vi "Voltage - Continuous Output.vi"() -> ()   [LabVIEW 2025]
doc: "This example demonstrates how to continuously re-generate analog output data from a buffer in your computer's memory.\n\nRefer to your device documentation for pinouts and hardware capabilities."
uses:
  <vilib>/Utility/error.llb/DialogType.ctl
  <vilib>/DAQmx/write.llb/DAQmx Write (Analog Wfm 1Chan NSamp).vi
  <vilib>/DAQmx/create/channels.llb/DAQmx Create Channel (AO-Voltage-Basic).vi
  <vilib>/DAQmx/configure/timing.llb/DAQmx Timing (Use Waveform).vi
  <vilib>/DAQmx/miscellaneous.llb/DAQmx Fill In Error Info.vi
panel:
  in  "Stop":bool
  out "Waveform Graph":waveform(dbl)(graph)
  in  "Max Voltage":dbl=5.0
  in  "Min Voltage":dbl=-5.0
  in  "Physical Channel(s)":tag="Dev1/ao0"
  # "Channel Settings"
  # "Output"
  # "Timing and\nBuffer Settings"
  # "Waveform Settings"
  # "The number of elements in the waveform array must equal the number of channels in the task."
  # "Trigger Settings"
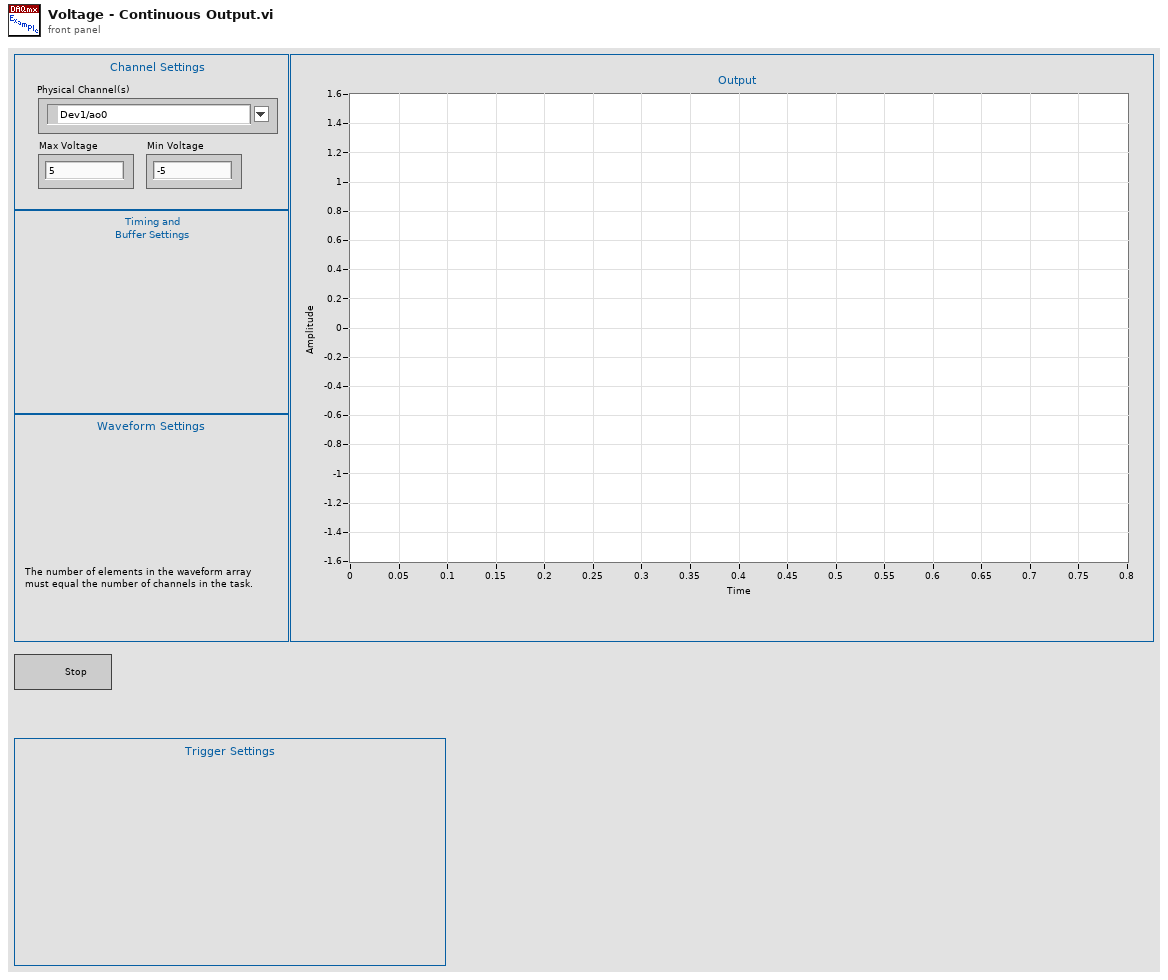
[diagram p1: front panel]
types:
  T1 = typedef "DialogType.ctl" = u16
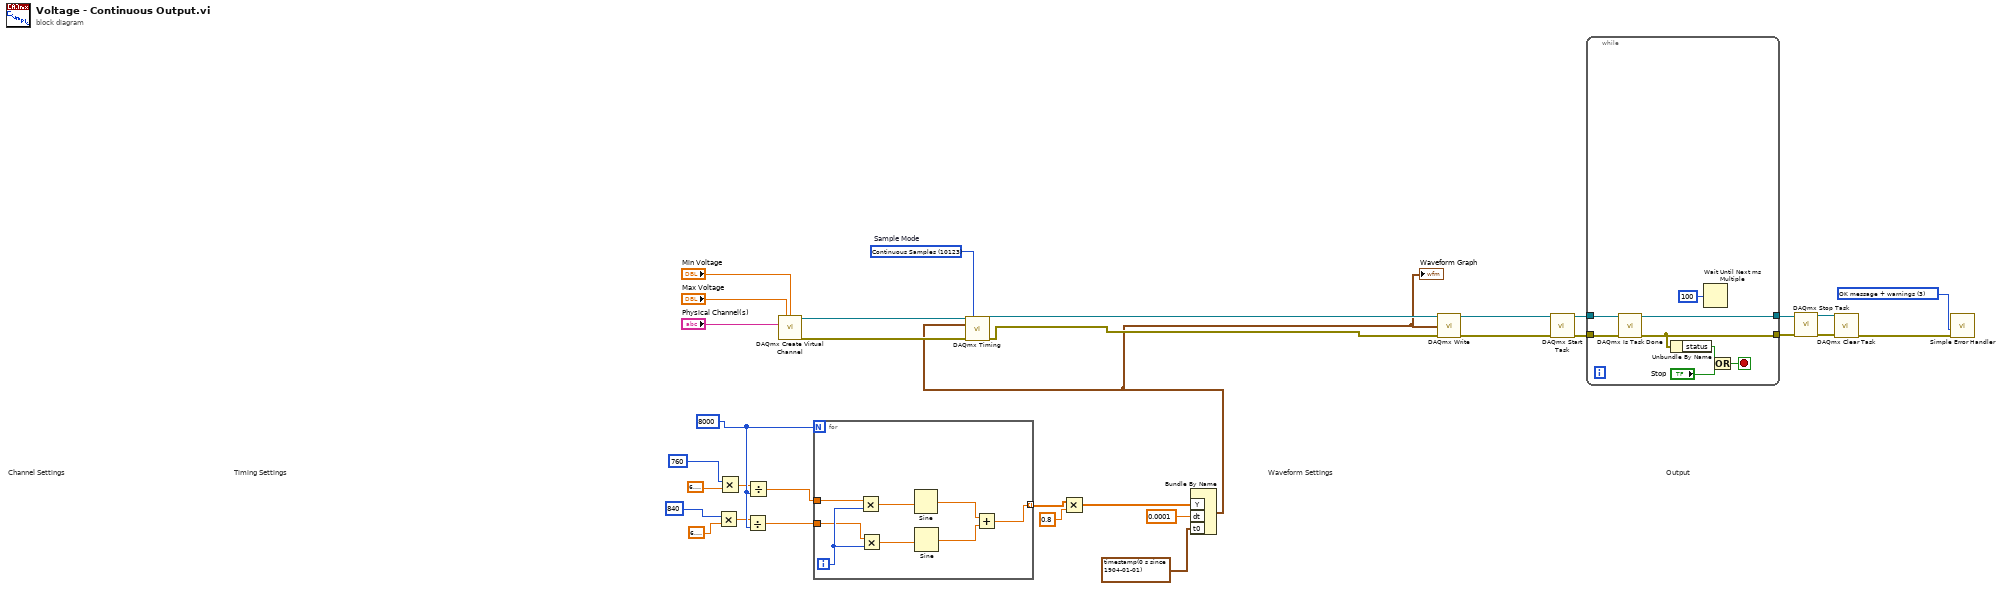
[diagram p0: block diagram]
diagram:
  w14 = 8000
  w18 = T1 3 items=["no dialog", "OK message", "continue or stop message", "OK message + warnings", "continue/stop + warnings"] ("type of dialog (OK msg:1)")
  w33 = 10123 items=["Finite Samples"=10178, "Continuous Samples"=10123, "Hardware Timed Single Point"=12522]  # Sample Mode
  # "Output"
  # "Waveform Settings"
  # "Timing Settings"
  # "Channel Settings"
  n1 = Multiply(x=840, y=6.283185307179586) -> (x*y=w12:dbl)
  n2 = Multiply(x=760, y=6.283185307179586) -> (x*y=w13:dbl)
  n3 = Divide(x=w12, y=w14) -> (x/y=w10:dbl)
  n4 = Divide(x=w13, y=w14) -> (x/y=w11:dbl)
  n5 = call-poly <vilib>:"DAQmx Create Virtual Channel.vi"("maximum value"="Max Voltage", "minimum value"="Min Voltage", "physical channels"="Physical Channel(s)") -> ("task out"=w31:refnum<k21>, "error out"=w32:errorcluster)  [unwired: 11 in]
  n6 = for {
    N: w14 -> [_]
    tunnel: [w34] -> w5 mode=indexing
    tunnel: w11 -> [w39]
    tunnel: w10 -> [w37]
    i -> [w38]
    n7 = Multiply(x=w39, y=w38) -> (x*y=w41:dbl)
    n8 = Multiply(x=w37, y=w38) -> (x*y=w40:dbl)
    n9 = Sine(x=w41) -> (sin(x)=w36:dbl)
    n10 = Sine(x=w40) -> (sin(x)=w35:dbl)
    n11 = Add(x=w36, y=w35) -> (x+y=w34:dbl)
  }
  n12 = Multiply(x=w5, y=0.8) -> (x*y=w3:dbl[])
  n13 = Bundle By Name("Y"=w3, "dt"=0.0001, "t0"=timestamp(0 s since 1904-01-01)) -> (w1:waveform(dbl))  [unwired: 1 in]
  "Waveform Graph" <- w1
  n14 = call-poly <vilib>:"DAQmx Timing.vi"("task/channels in"=w31, "sample mode"=w33, "waveform"=w1, "error in"=w32) -> ("task out"=w17:refnum<k21>, "error out"=w16:errorcluster)  [unwired: 10 in]
  n15 = call-poly <vilib>:"DAQmx Write.vi"("task/channels in"=w17, "data"=w1, "error in"=w16) -> ("task out"=w24:refnum<k21>, "error out"=w23:errorcluster)  [unwired: 10 in, 1 out]
  n16 = call <vilib>:"DAQmx Start Task.vi"("task/channels in"=w24, "error in"=w23) -> ("task out"=w30:refnum<k21>, "error out"=w29:errorcluster)  [unwired: 12 in]
  n17 = while {
    tunnel: w30 -> [w49]
    tunnel: w29 -> [w48]
    tunnel: [w45] -> w19
    tunnel: [w46] -> w20
    stop <- w47 stop-if-true
    n18 = call <vilib>:"DAQmx Is Task Done.vi"("task/channels in"=w49, "error in"=w48) -> ("task out"=w46:refnum<k21>, "error out"=w45:errorcluster)  [unwired: 11 in, 1 out]
    n19 = Unbundle By Name(w45) -> ("status"=w44:bool)
    n20 = Wait Until Next ms Multiple(millisecond multiple=u32 100) -> ()  [unwired: 1 out]
    n21 = Or(x=w44, y="Stop") -> (x .or. y?=w47:bool)
  }
  n22 = call <vilib>:"DAQmx Stop Task.vi"("task/channels in"=w20, "error in"=w19) -> ("task out"=w22:refnum<k21>, "error out"=w21:errorcluster)  [unwired: 12 in]
  n23 = call <vilib>:"DAQmx Clear Task.vi"("task in"=w22, "error in"=w21) -> ("error out"=w28:errorcluster)  [unwired: 13 in]
  n24 = call <vilib>:"Simple Error Handler.vi"("type of dialog (OK msg:1)"=w18, "error in (no error)"=w28) -> ()  [unwired: 3 in, 5 out]
